vi "Set FPGA target.vi"(8 "error in (no error)":errorcluster, 10 "Number of bits":i32, 11 "Boolean array":bool[](array[boolean])) -> (0 "error out":errorcluster)   [LabVIEW 2013]
uses:
  <vilib>/DAQmx/write.llb/DAQmx Write (Digital Bool 1Line 1Point).vi
  <vilib>/DAQmx/miscellaneous.llb/DAQmx Fill In Error Info.vi
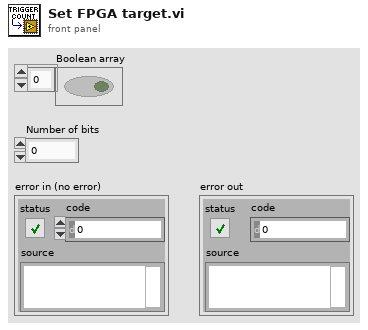
[diagram p1: front panel]
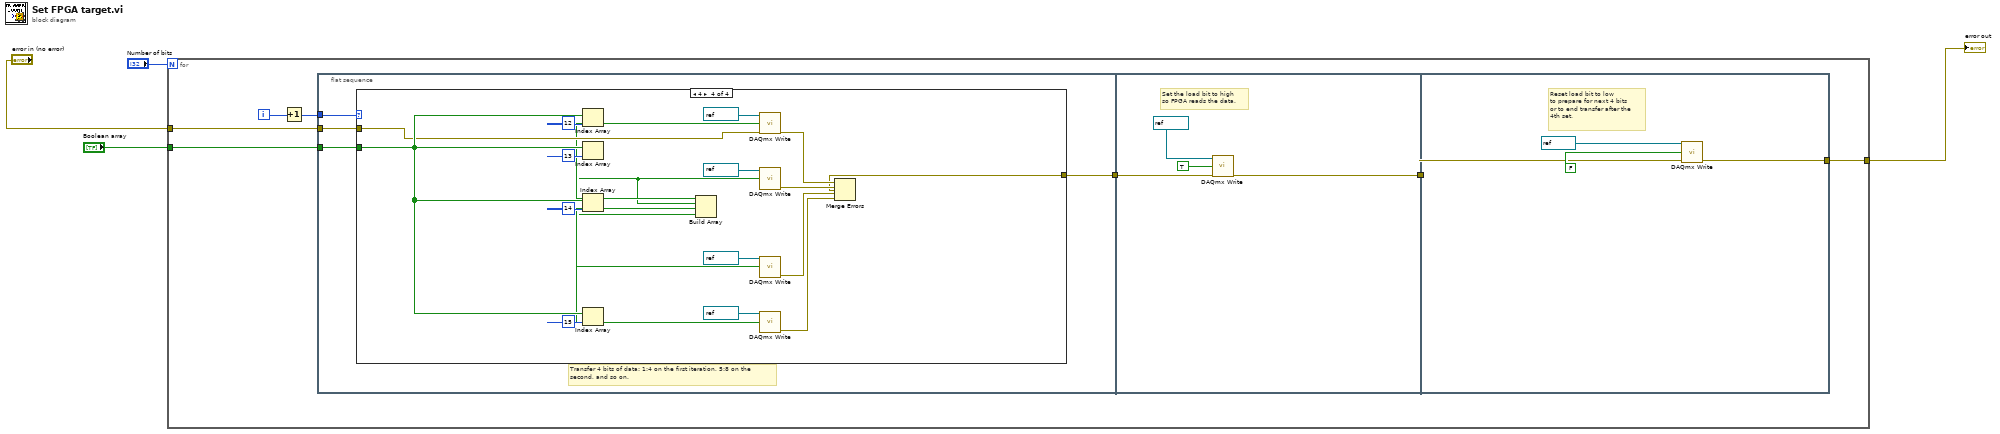
[diagram p0: block diagram]
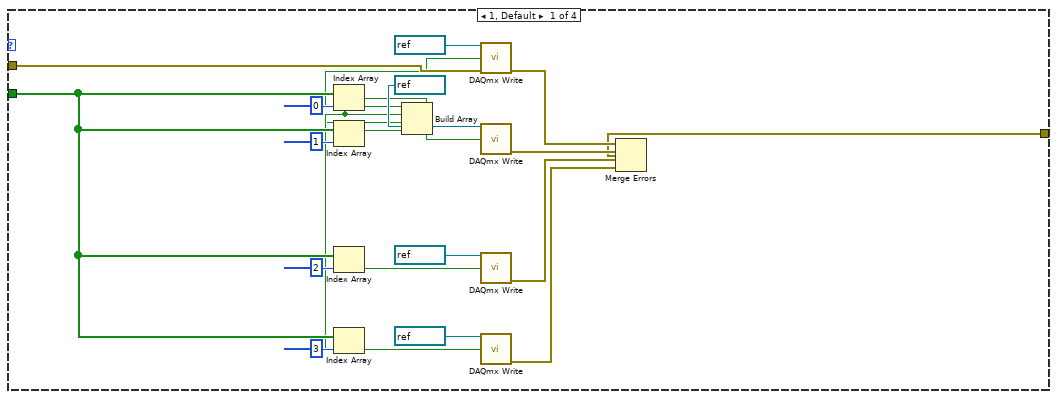
[diagram p2: hidden frame]
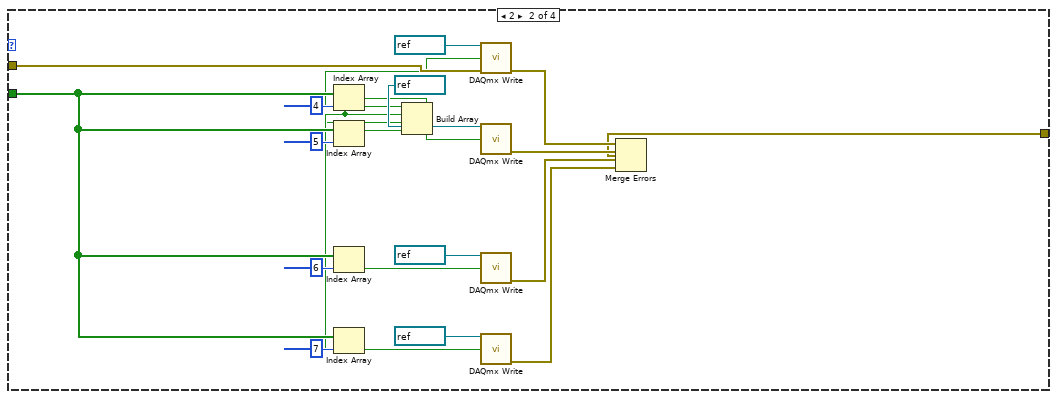
[diagram p3: hidden frame]
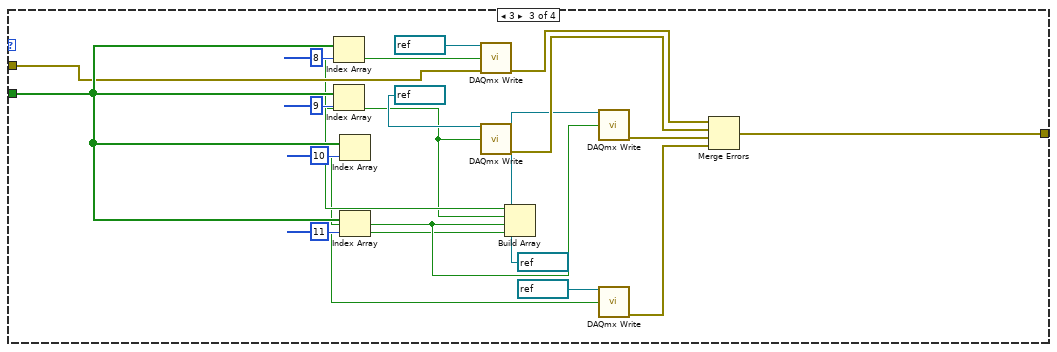
[diagram p4: hidden frame]
diagram:
  n1 = for {
    N: "Number of bits" -> [_]
    tunnel: "Boolean array" -> [w8]
    tunnel: "error in (no error)" -> [w10]
    tunnel: [w5] -> w4
    i -> [w11]
    n2 = Increment(x=w11) -> (x+1=w9:i32)
    n3 = flat-sequence {
      tunnel: w10 -> [w15]
      tunnel: w9 -> [w14]
      tunnel: w8 -> [w13]
      tunnel: [w12] -> w7
      tunnel: w7 -> [w93]
      tunnel: [w92] -> w6
      tunnel: w6 -> [w97]
      tunnel: [w96] -> w5
      frame #0 {
        # "Transfer 4 bits of data: 1:4 on the first iteration, 5:8 on the\nsecond, and so on."
        n4 = case shown="4" w14 {
          tunnel: w13 -> [w22 w41 w60 w79]
          tunnel: w15 -> [w21 w40 w59 w78]
          tunnel: [w20 w39 w58 w77] -> w12
          frame 1, Default {
            n5 = Index Array(array=w22, index=0) -> (element=w19:bool)
            n6 = Index Array(array=w22, index=1) -> (element=w18:bool)
            n7 = Index Array(array=w22, index=2) -> (element=w17:bool)
            n8 = Index Array(array=w22, index=3) -> (element=w16:bool)
            n9 = Build Array(w19, w18, w17, w16) -> ()  [unwired: 1 out]
            n10 = call-poly <vilib>:"DAQmx Write.vi"("task/channels in"=refnum<k21> "BIT1", "data"=w19, "error in"=w21) -> ("error out"=w30:errorcluster)  [unwired: 10 in, 2 out]
            n11 = call-poly <vilib>:"DAQmx Write.vi"("task/channels in"=refnum<k21> "BIT2", "data"=w18) -> ("error out"=w29:errorcluster)  [unwired: 11 in, 2 out]
            n12 = call-poly <vilib>:"DAQmx Write.vi"("task/channels in"=refnum<k21> "BIT3", "data"=w17) -> ("error out"=w28:errorcluster)  [unwired: 11 in, 2 out]
            n13 = call-poly <vilib>:"DAQmx Write.vi"("task/channels in"=refnum<k21> "BIT4", "data"=w16) -> ("error out"=w27:errorcluster)  [unwired: 11 in, 2 out]
            n14 = Merge Errors(w30, w29, w28, w27) -> (w20:errorcluster)
          }
          frame 2 {
            n15 = Index Array(array=w41, index=4) -> (element=w38:bool)
            n16 = Index Array(array=w41, index=5) -> (element=w37:bool)
            n17 = Index Array(array=w41, index=6) -> (element=w36:bool)
            n18 = Index Array(array=w41, index=7) -> (element=w35:bool)
            n19 = Build Array(w38, w37, w36, w35) -> ()  [unwired: 1 out]
            n20 = call-poly <vilib>:"DAQmx Write.vi"("task/channels in"=refnum<k21> "BIT1", "data"=w38, "error in"=w40) -> ("error out"=w49:errorcluster)  [unwired: 10 in, 2 out]
            n21 = call-poly <vilib>:"DAQmx Write.vi"("task/channels in"=refnum<k21> "BIT2", "data"=w37) -> ("error out"=w48:errorcluster)  [unwired: 11 in, 2 out]
            n22 = call-poly <vilib>:"DAQmx Write.vi"("task/channels in"=refnum<k21> "BIT3", "data"=w36) -> ("error out"=w47:errorcluster)  [unwired: 11 in, 2 out]
            n23 = call-poly <vilib>:"DAQmx Write.vi"("task/channels in"=refnum<k21> "BIT4", "data"=w35) -> ("error out"=w46:errorcluster)  [unwired: 11 in, 2 out]
            n24 = Merge Errors(w49, w48, w47, w46) -> (w39:errorcluster)
          }
          frame 3 {
            n25 = Index Array(array=w60, index=8) -> (element=w57:bool)
            n26 = Index Array(array=w60, index=9) -> (element=w56:bool)
            n27 = Index Array(array=w60, index=10) -> (element=w55:bool)
            n28 = Index Array(array=w60, index=11) -> (element=w54:bool)
            n29 = call-poly <vilib>:"DAQmx Write.vi"("task/channels in"=refnum<k21> "BIT1", "data"=w57, "error in"=w59) -> ("error out"=w68:errorcluster)  [unwired: 10 in, 2 out]
            n30 = call-poly <vilib>:"DAQmx Write.vi"("task/channels in"=refnum<k21> "BIT2", "data"=w56) -> ("error out"=w67:errorcluster)  [unwired: 11 in, 2 out]
            n31 = Build Array(w57, w56, w55, w54) -> ()  [unwired: 1 out]
            n32 = call-poly <vilib>:"DAQmx Write.vi"("task/channels in"=refnum<k21> "BIT3", "data"=w55) -> ("error out"=w66:errorcluster)  [unwired: 11 in, 2 out]
            n33 = call-poly <vilib>:"DAQmx Write.vi"("task/channels in"=refnum<k21> "BIT4", "data"=w54) -> ("error out"=w65:errorcluster)  [unwired: 11 in, 2 out]
            n34 = Merge Errors(w68, w67, w66, w65) -> (w58:errorcluster)
          }
          frame 4 {
            n35 = Index Array(array=w79, index=12) -> (element=w76:bool)
            n36 = Index Array(array=w79, index=13) -> (element=w75:bool)
            n37 = Index Array(array=w79, index=14) -> (element=w74:bool)
            n38 = Index Array(array=w79, index=15) -> (element=w73:bool)
            n39 = Build Array(w76, w75, w74, w73) -> ()  [unwired: 1 out]
            n40 = call-poly <vilib>:"DAQmx Write.vi"("task/channels in"=refnum<k21> "BIT1", "data"=w76, "error in"=w78) -> ("error out"=w87:errorcluster)  [unwired: 10 in, 2 out]
            n41 = call-poly <vilib>:"DAQmx Write.vi"("task/channels in"=refnum<k21> "BIT2", "data"=w75) -> ("error out"=w86:errorcluster)  [unwired: 11 in, 2 out]
            n42 = call-poly <vilib>:"DAQmx Write.vi"("task/channels in"=refnum<k21> "BIT3", "data"=w74) -> ("error out"=w85:errorcluster)  [unwired: 11 in, 2 out]
            n43 = call-poly <vilib>:"DAQmx Write.vi"("task/channels in"=refnum<k21> "BIT4", "data"=w73) -> ("error out"=w84:errorcluster)  [unwired: 11 in, 2 out]
            n44 = Merge Errors(w87, w86, w85, w84) -> (w77:errorcluster)
          }
        }
      }
      frame #1 {
        # "Set the load bit to high\nso FPGA reads the data."
        n45 = call-poly <vilib>:"DAQmx Write.vi"("task/channels in"=refnum<k21> "BIT5", "data"=TRUE, "error in"=w93) -> ("error out"=w92:errorcluster)  [unwired: 10 in, 2 out]
      }
      frame #2 {
        # "Reset load bit to low\nto prepare for next 4 bits\nor to end transfer after the\n4th set."
        n46 = call-poly <vilib>:"DAQmx Write.vi"("task/channels in"=refnum<k21> "BIT5", "data"=FALSE, "error in"=w97) -> ("error out"=w96:errorcluster)  [unwired: 10 in, 2 out]
      }
    }
  }
  "error out" <- w4
